vi "Configure AUX Measurement.vi"(0 "VISA resource name":refnum<visa-resource-name>, 1 "Channel (1)":i32=1, 2 "Port (1)":i32=1, 3 "Trace (1)":i32=1, 9 "Measurement Parameter (0:AUX1)":u16(ring) items=["AUX1", "AUX2"], 11 "error in (no error)":errorcluster, 12 "AUX DC Input Range (10)":dbl=10.0) -> (4 "VISA resource name out":refnum<visa-resource-name>, 15 "error out":errorcluster)   [LabVIEW 2011, in "Agilent ENA Series.lvlib"]
doc: "This VI configures AUX measurement of active channel.\n\nNotes:\n(1) Only E5071C supports AUX measurement."
uses:
  Agilent ENA Series.lvlib
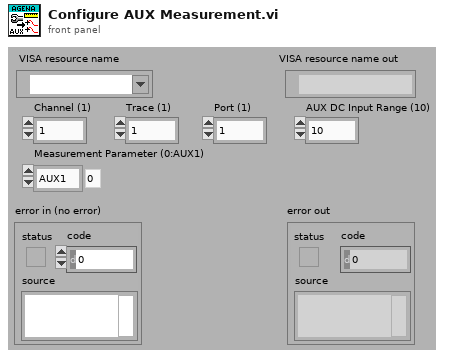
[diagram p1: front panel]
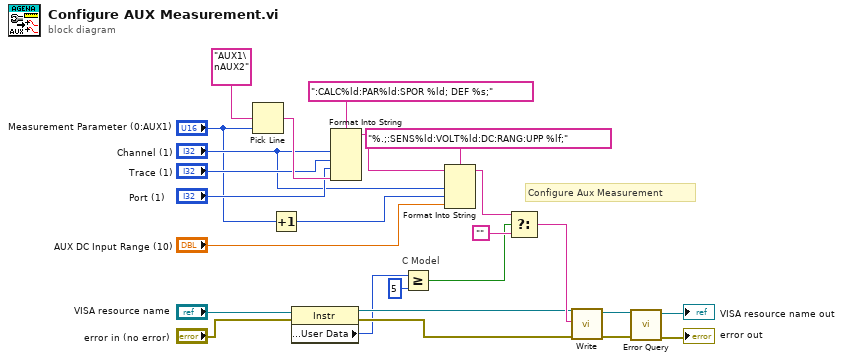
[diagram p0: block diagram]
diagram:
  # "Configure Aux Measurement"
  # "C Model"
  n1 = Pick Line(multi-line string="AUX1\nAUX2", line index="Measurement Parameter (0:AUX1)") -> (output string=w23:string)  [unwired: 1 in]
  n2 = Increment(x="Measurement Parameter (0:AUX1)") -> (x+1=w10:u16)
  n3 = property class="Instr"(reference="VISA resource name", error in="error in (no error)") -> (reference out=w6:refnum<visa-resource-name>, error out=w5:errorcluster, "General Settings:User Data"=w3:u32)
  n4 = Format Into String(format string=":CALC%ld:PAR%ld:SPOR %ld; DEF %s;", "Channel (1)", "Trace (1)", "Port (1)", w23) -> (resulting string=w12:string)  [unwired: 2 in, 1 out]
  n5 = Greater Or Equal?(x=w3, y=u32 5) -> (x >= y?=w2:bool)
  n6 = Format Into String(format string="%.;:SENS%ld:VOLT%ld:DC:RANG:UPP %lf;", initial string=w12, "Channel (1)", w10, "AUX DC Input Range (10)") -> (resulting string=w13:string)  [unwired: 1 in, 1 out]
  n7 = Select(t=w13, s=w2, f="") -> (s? t:f=w11:string)
  n8 = call "Write.vi"("error in (no error)"=w5, "String ()"=w11, "VISA resource name"=w6) -> ("error out"=w19:errorcluster, "VISA resource name out"=w20:refnum<visa-resource-name>)  [unwired: 6 in, 1 out]
  n9 = call "Error Query.vi"("error in (no error)"=w19, "VISA resource name"=w20) -> ("error out"=→"error out":errorcluster, "VISA resource name out"=→"VISA resource name out":refnum<visa-resource-name>)  [unwired: 6 in, 2 out]
